vi "CleanUpNode.vi"(8 "error in":errorcluster, 10 "Parameters":variant, 11 "TEC editor node in":refnum<class "TEC editor node.lvclass">) -> (0 "error out":errorcluster, 3 "TEC editor node out":refnum<class "TEC editor node.lvclass">)   [LabVIEW 2013, in "TEC editor node.lvclass"]
doc: "This VI will clean any reference handled internally in the node"
uses:
  TEC editor node.lvclass
  <vilib>/NI/Tag Bus Data Framework/Configuration Editor/Classes/Module editor node/module editor node.lvclass
  <vilib>/NI/Tag Bus Data Framework/Configuration Editor/Classes/Engine Parent/Engine Parent Editor Node.lvclass
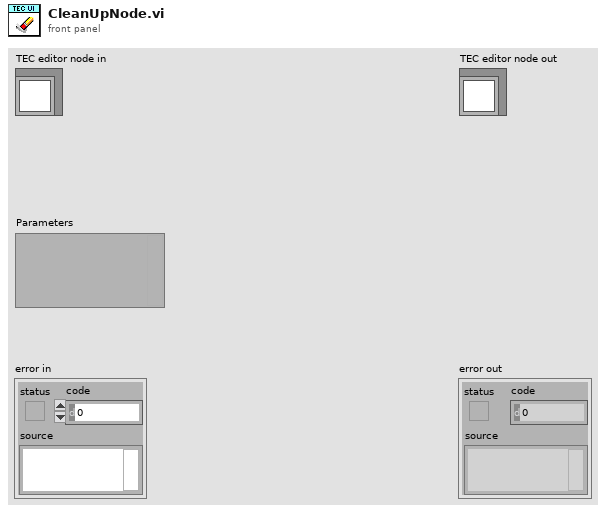
[diagram p1: front panel]
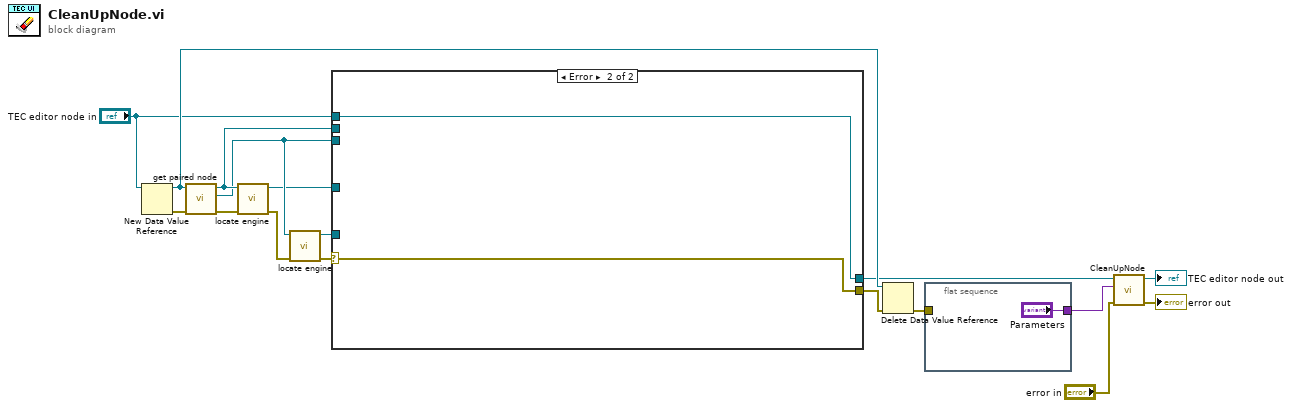
[diagram p0: block diagram]
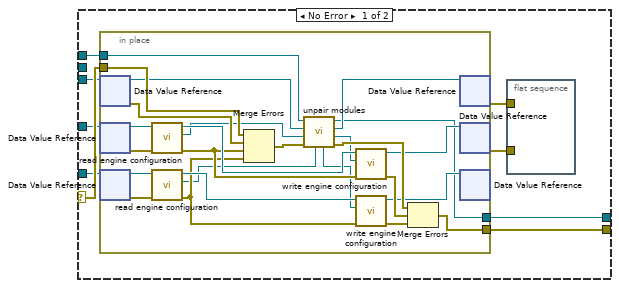
[diagram p2: hidden frame]
diagram:
  n1 = New Data Value Reference(data value="TEC editor node in") -> (data value reference=w13:refnum<data-value>, error out=w15:errorcluster)  [unwired: 1 in]
  n2 = call "get paired node.vi"("error in"=w15, "editor in"=w13) -> ("error out"=w8:errorcluster, "paired node"=w6:refnum<data-value>, "editor out"=w9:refnum<data-value>)  [unwired: 7 in]
  n3 = call <vilib>:"locate engine.vi"("error in"=w8, "component"=w9) -> ("error out"=w7:errorcluster, "engine"=w3:refnum<data-value>)  [unwired: 8 in]
  n4 = call <vilib>:"locate engine.vi"("error in"=w7, "component"=w6) -> ("error out"=w5:errorcluster, "engine"=w4:refnum<data-value>)  [unwired: 8 in]
  n5 = case shown="Error" w5 {
    selector: w5 -> [w24 w53]
    tunnel: [w23 w53] -> w14
    tunnel: w9 -> [_ _]
    tunnel: w6 -> [w20 _]
    tunnel: w4 -> [w22 _]
    tunnel: w3 -> [w21 _]
    tunnel: "TEC editor node in" -> [w19 w52]
    tunnel: [w18 w52] -> w1
    frame No Error {
      n6 = in-place {
        in-place-border: w24 -> [w51]
        in-place-border: [w39] -> w23
        in-place-border: w19 -> [w28]
        in-place-border: [w27] -> w18
        n7 = in-place-dvr #1(w20) -> (w49:refnum<class "TEC editor node.lvclass">, w47:errorcluster)
        n8 = in-place-dvr #2(w21) -> (w45:refnum<class "Engine Parent Editor Node.lvclass">, w44:errorcluster)
        n9 = in-place-dvr #3(w22) -> (w35:refnum<class "Engine Parent Editor Node.lvclass">, w34:errorcluster)
        n10 = call <vilib>:"read engine configuration.vi"("error in"=w44, "Engine Parent Editor Node in"=w45) -> ("error out"=w37:errorcluster, "engine configuration"=w41:refnum<class "engine configuration.lvclass">, "Engine Parent Editor Node out"=w43:refnum<class "Engine Parent Editor Node.lvclass">)  [unwired: 7 in]
        n11 = call <vilib>:"read engine configuration.vi"("error in"=w34, "Engine Parent Editor Node in"=w35) -> ("error out"=w33:errorcluster, "engine configuration"=w29:refnum<class "engine configuration.lvclass">, "Engine Parent Editor Node out"=w36:refnum<class "Engine Parent Editor Node.lvclass">)  [unwired: 7 in]
        n12 = Merge Errors(w51, w47, w37, w33) -> (w48:errorcluster)
        n13 = call "unpair modules.vi"("paired engine in"=w29, "error in"=w48, "engine configuration in"=w41, "module to unpair"=w49, "UDP Broadcast Editor Node in"=w28) -> ("error out"=w50:errorcluster, "engine configuration out"=w40:refnum<class "engine configuration.lvclass">, "unpaired module"=w46:refnum<class "TEC editor node.lvclass">, "UDP Broadcast Editor Node out"=w27:refnum<class "TEC editor node.lvclass">, "paired engine out"=w30:refnum<class "engine configuration.lvclass">)  [unwired: 2 in]
        n14 = call <vilib>:"write engine configuration.vi"("error in"=w37, "engine configuration"=w40, "Engine Parent Editor Node in"=w43) -> ("error out"=w38:errorcluster, "Engine Parent Editor Node out"=w42:refnum<class "Engine Parent Editor Node.lvclass">)  [unwired: 7 in]
        n15 = call <vilib>:"write engine configuration.vi"("error in"=w33, "engine configuration"=w30, "Engine Parent Editor Node in"=w36) -> ("error out"=w32:errorcluster, "Engine Parent Editor Node out"=w31:refnum<class "Engine Parent Editor Node.lvclass">)  [unwired: 7 in]
        n16 = Merge Errors(w50, w38, w32) -> (w39:errorcluster)
        n17 = in-place-dvr #1(w46) -> (w25:errorcluster)  [unwired: 1 out]
        n18 = in-place-dvr #2(w42) -> (w26:errorcluster)  [unwired: 1 out]
        n19 = in-place-dvr #3(w31) -> ()  [unwired: 2 out]
      }
      n20 = flat-sequence {
        tunnel: w25 -> [_]
        tunnel: w26 -> [_]
        frame #0 {
        }
      }
    }
    frame Error {
    }
  }
  n21 = Delete Data Value Reference(data value reference=w13, error in=w14) -> (error out=w10:errorcluster)  [unwired: 1 out]
  n22 = flat-sequence {
    tunnel: ["Parameters"] -> w16
    tunnel: w10 -> [_]
    frame #0 {
    }
  }
  n23 = call-parent "CleanUpNode.vi"("error in"="error in", "Parameters"=w16, "module editor node in"=w1) -> ("error out"=→"error out":errorcluster, "module editor node out"=→"TEC editor node out":refnum<class "TEC editor node.lvclass">)  [unwired: 7 in]
